vi "Build.vi"(8 "error in (no error)":errorcluster, 11 "Build in":refnum<class "AB_RESTfulWebService.lvclass">) -> (0 "error out":errorcluster, 1 "GeneratedFiles":path[](array[path]), 2 "GeneratedDirectories":path[](array[path]), 3 "Build out":refnum<class "AB_RESTfulWebService.lvclass">, 4 "GeneratedFileGUIDs":string[](array[string]), 5 "OutputDirectory":path, 7 "Dependencies":T1[](array[typedef]))   [LabVIEW 2020, in "AB_RESTfulWebService.lvclass"]
uses:
  <vilib>/AppBuilder/AB_Classes/RESTful/AB_RESTfulWebService.lvclass
  e:/builds/penguin/labview/branches/2020/dev/dist/vi.lib/AppBuilder/AB_Classes/Build/AB_Build.lvclass
  e:/builds/penguin/labview/branches/2020/dev/dist/vi.lib/AppBuilder/AB_Classes/TargetFile/AB_Targetfile.lvclass
  e:/builds/penguin/labview/branches/2020/dev/dist/vi.lib/AppBuilder/AB_Classes/WebService/AB_WebService.lvclass
  <vilib>/AppBuilder/AB_Dependency.ctl
  <vilib>/Utility/lvfile.llb/LVFileType.ctl
  <vilib>/AppBuilder/Engine/RESTful INI Generator/AB_RESTful_ServiceType.ctl
  <vilib>/AppBuilder/Engine/RESTful INI Generator/AB_RESTful_ServiceInfo.ctl
  <vilib>/AppBuilder/AB_Classes/RESTful/AB_RESTful_ServiceAttribute.ctl
  <vilib>/AppBuilder/AB_Classes/RESTful/AB_RESTful_ServiceAttributeType.ctl
  <vilib>/AppBuilder/AB_Classes/RESTful/AB_RESTfulWebService.lvclass/AB_RESTfulWebService.ctl
  <resource>/Framework/Providers/Common/provcom_StringGlobals.vi
  <vilib>/AppBuilder/AB_Classes/WebService/AB_WebService.lvclass
  <vilib>/AppBuilder/AB_Classes/Destination/AB_Destination.lvclass
  <vilib>/AppBuilder/AB_Classes/Build/AB_Build.lvclass
  <vilib>/AppBuilder/AB_Classes/TargetFile/AB_Targetfile.lvclass
  <vilib>/Utility/lvfile.llb/NI_FileType.lvlib
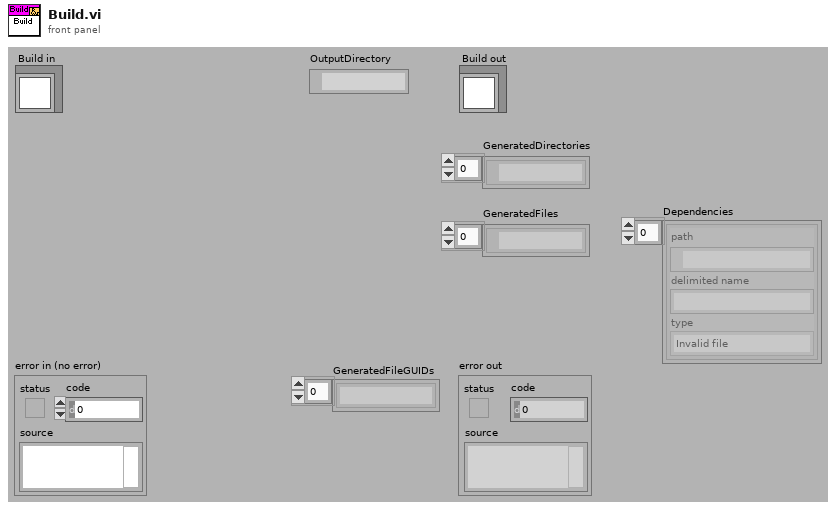
[diagram p1: front panel]
types:
  T1 = typedef "AB_Dependency.ctl" = cluster{"path":path, "delimited name":string, "type":T2}
  T2 = typedef "NI_FileType.lvlib/LVFileType.ctl" = enum32{"Invalid file", "Unknown type", "Instrument", "Control", "Polymorphic VI", "Project", "Library", "LVClass", "XControl", "XNode", "Shared library", ".NET assembly", "ActiveX interface", "CIN", "Run-time menu", "Palette menu", "Help file", "LLB", "XNode Edit Dependency", "Class Private Data Control", "Statechart", "MathScript .m file", "Ladder Diagram", "LVLibp", "XNode Build Dependency"}
  T3 = typedef "AB_RESTful_ServiceInfo.ctl" = cluster{"Service Name":string, "Web Service Library Path":path, "Server List":string[], "Debug":bool, "Service aliases":string[], "defaultStaticDoc":string, "defaultWebMethod":string, "Standalone":bool, "Service attributes":T4[], "Service Type":T6, "IniVersion":string, "MessageVersion":string, "RoutingKey":string, "Type":string, "Tags":string}
  T4 = typedef "AB_RESTful_ServiceAttribute.ctl" = cluster{"Name":string, "Service Attribute Type":T5, "Value":string}
  T5 = typedef "AB_RESTful_ServiceAttributeType.ctl" = enum32{"String", "Path"}
  T6 = typedef "AB_RESTful_ServiceType.ctl" = enum32{"RESTful", "SOAP", "AMQP"}
  T7 = typedef "AB_Build.ctl" = cluster{"buildSpecName":string, "buildSpecDescription":string, "destinations":refnum<class "AB_Destination.lvclass">[], "exclusionOption":T8, "defaultLanguage":string, "supportedLanguages":string[], "excludedDirectories":path[], "buildContext":refnum<vi>, "buildObject":T9, "preview":bool, "programatic":bool, "progressBarEvents":T10, "userLog_Path":path, "preActionID":string, "preAction_Path":path, "postActionID":string, "postAction_Path":path, "eng_checkForBrokenVIs?":bool, "eng_verboseLinkerErrors?":bool, "localDest_Path":path, "targetDest_Path":path, "removeVIObject":u16, "cache":refnum<class "PreviewCache.lvclass">, "use cache":bool, "previewCache_ID":string, "buildCache_ID":string, "eng_TempLocalDest_Path":path, "eng_collectDependencies?":bool, "versionInfo":cluster{"buildVersion":cluster{"major":u16, "minor":u16, "patch":u16, "build":u16}, "autoIncrement":bool}, "eng_enableVIChecksums":bool}
  T8 = typedef "AB_Exclusion_Option.ctl" = cluster{"typedefs":bool, "polymorphicVIs":bool, "unusedLibraryItems":bool, "modifyLibraryFile":bool, "edit-timeDependencies":bool, "inlineVIs":bool, "dependent PPLs":bool, "dependent DLLs":bool}
  T9 = typedef "ItemRef.ctl" = u64
  T10 = typedef "provcom_ProgressBar_Events.ctl" = cluster{"newJob":refnum<user-event>, "newItem":refnum<user-event>, "errorMsg":T11, "cancel":refnum<user-event>}
  T11 = typedef "mxLvBuildError.ctl" = refnum<user-event>
  T12 = typedef "AB_RESTful_RoutingTemplate.ctl" = cluster{"Template":string, "Routing Type":T13, "HTTP Method Type":T14, "VIName":string, "Default String":string, "Require API key":bool, "Auth permissions":string[], "eng_Static Alias":string, "Required Privilege":string}
  T13 = typedef "AB_RESTful_RoutingType.ctl" = enum32{"Method", "Static"}
  T14 = typedef "AB_RESTful_HTTPMethodType.ctl" = enum32{"GET", "POST", "PUT", "DELETE"}
  T15 = cluster{"Privilege":string, "Description":string, "Role":string}[]
  T16 = typedef "AB_Targetfile.ctl" = cluster{"targetfileName":string, "targetfileGUID":string, "enableDebugging":bool, "versionInfo":cluster{"productName":string, "legalCopyright":string, "companyName":string, "internalName":string, "fileDescription":string}, "eng_consolidatedTypeInfo":string, "fastFileFormat":bool, "eng_LEIFBuildData":u32, "versionIndependent":bool}
  T17 = typedef "AB_WebService.ctl" = cluster{"service aliases":string[], "standalone":bool}
  T18 = typedef "AB_Destination.ctl" = cluster{"destName":string, "path":path, "libraryName":string, "preserveHierarchy":bool, "eng_inBuild":bool, "eng_libraryReference":refnum<vi>, "eng_restictAddToNewLibrary":bool}
  T19 = typedef "AB_RESTful_Configuration.ctl" = cluster{"Service VI Type":T20, "Load VI at statup":bool, "Keep VI in memory":bool, "Output type":T21, "Output format":T22, "Use headers":bool, "Buffered":bool, "eng_Load VI by name":bool}
  T20 = typedef "AB_RESTful_VIType.ctl" = enum32{"Web Method", "Auxiliary", "eng_Internal", "eng_Content"}
  T21 = typedef "AB_RESTful_OutputType.ctl" = enum32{"Terminal", "Stream"}
  T22 = typedef "AB_RESTful_OutputFormat.ctl" = enum32{"XML", "Text", "HTML", "JSON"}
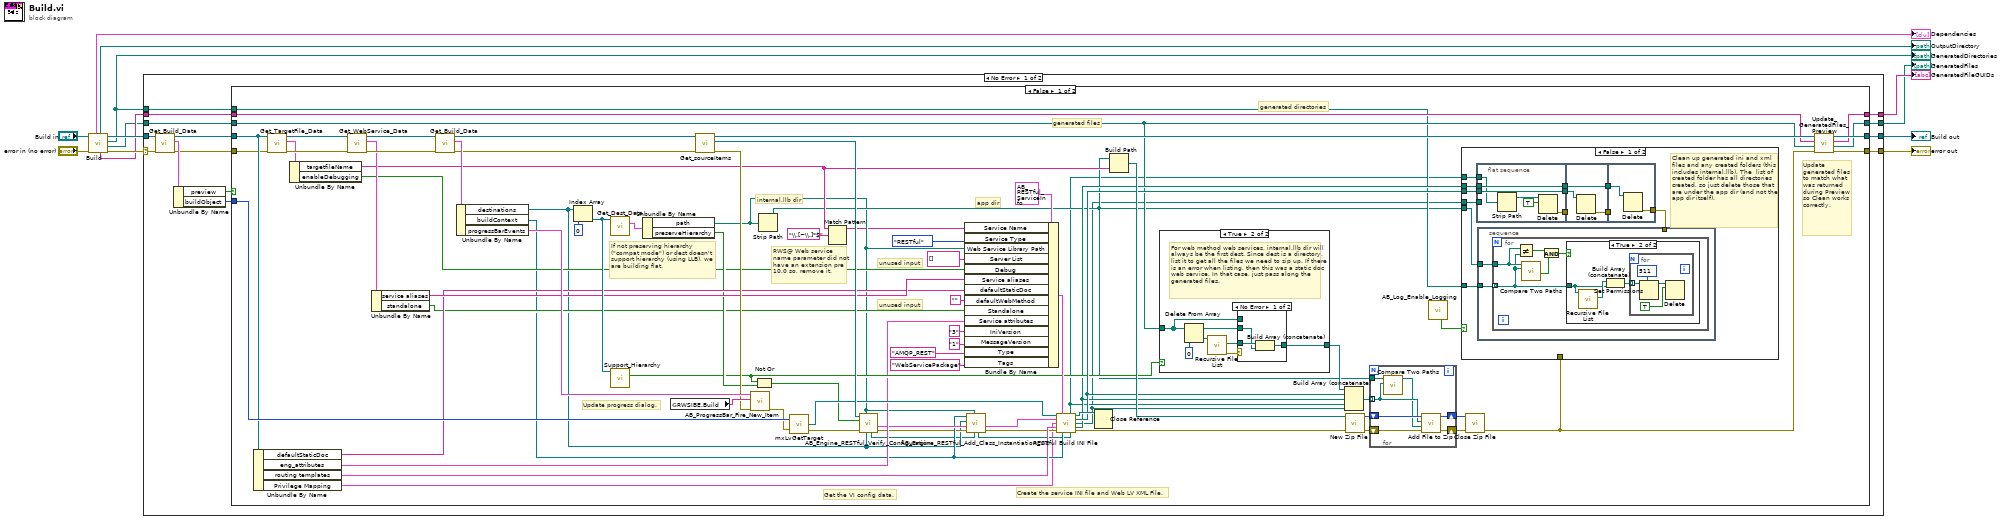
[diagram p0: block diagram]
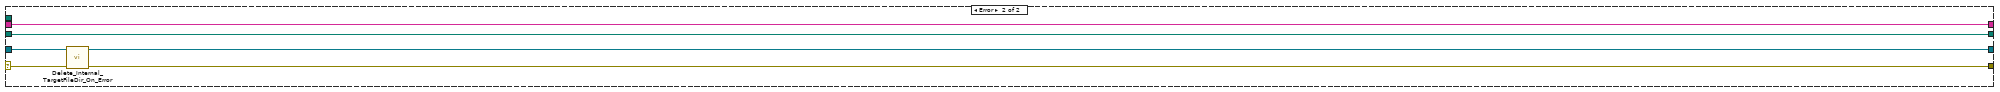
[diagram p7: hidden frame]
diagram:
  n1 = call-parent "Build.vi"("error in (no error)"="error in (no error)", "Build in"="Build in") -> ("error out"=w10:errorcluster, "GeneratedFiles"=w4:path[], "GeneratedDirectories"=w2:path[], "Build out"=w9:refnum<class "AB_RESTfulWebService.lvclass">, "GeneratedFileGUIDs"=w6:string[], "OutputDirectory"=→"OutputDirectory":path, "Dependencies"=→"Dependencies":T1[])  [unwired: 3 out]
  "GeneratedDirectories" <- w2
  n2 = case shown="No Error" w10 {
    selector: w10 -> [w25 w169]
    tunnel: w9 -> [w26 w170]
    tunnel: [w21 w167] -> w8
    tunnel: [w20 w168] -> w7
    tunnel: w4 -> [w18 w166]
    tunnel: w6 -> [w17 w165]
    tunnel: [w16 w165] -> w5
    tunnel: [w15 w166] -> w3
    tunnel: w2 -> [w14 _]
    frame No Error {
      n3 = call <vilib>:"Get_Build_Data.vi"("error in (no error)"=w25, "Class in"=w26) -> ("error out"=w23:errorcluster, "data"=w27:T7, "Class out"=w22:refnum<class "AB_RESTfulWebService.lvclass">)  [unwired: 7 out]
      n4 = Unbundle By Name(w27) -> ("preview"=w24:bool, "buildObject"=w19:T9)
      n5 = case shown="False" w24 {
        tunnel: w23 -> [w64 w163]
        tunnel: w22 -> [w66 w164]
        tunnel: [w53 w164] -> w21
        tunnel: [w55 w163] -> w20
        tunnel: w19 -> [w92 _]
        tunnel: w18 -> [w52 w162]
        tunnel: w17 -> [w51 w161]
        tunnel: [w50 w161] -> w16
        tunnel: [w49 w162] -> w15
        tunnel: w14 -> [w48 _]
        frame False {
          # "generated directories"
          # "Update generated files to match what was returned during Preview so Clean works correctly."
          # "unused input"
          # "RWS@ Web service name parameter did not have an extension pre 10.0 so, remove it."
          # "unused input"
          # "If not preserving hierarchy (\"compat mode\") or dest doesn't support hierarchy (using LLB), we are building flat."
          # "generated files"
          # "Update progress dialog."
          # "Create the service INI file and Web LV XML File."
          # "Get the VI config data."
          # "app dir"
          # "internal.llb dir"
          n6 = Unbundle By Name(w66) -> ("defaultStaticDoc"=w80:string, "eng_attributes"=w46:T4[], "routing templates"=w96:T12[], "Privilege Mapping"=w31:T15)
          n7 = call <vilib>:"Get_TargetFile_Data.vi"("error in (no error)"=w64, "AB_Targetfile in"=w66) -> ("error out"=w63:errorcluster, "data"=w62:T16, "AB_Targetfile out"=w65:refnum<class "AB_RESTfulWebService.lvclass">)  [unwired: 7 in]
          n8 = Unbundle By Name(w62) -> ("targetfileName"=w59:string, "enableDebugging"=w61:bool)
          n9 = call <vilib>:"Get_WebService_Data.vi"("error in (no error)"=w63, "Class in"=w65) -> ("error out"=w100:errorcluster, "data"=w99:T17, "class out"=w101:refnum<class "AB_RESTfulWebService.lvclass">)  [unwired: 7 out]
          n10 = Unbundle By Name(w99) -> ("service aliases"=w81:string[], "standalone"=w57:bool)
          n11 = call <vilib>:"Get_Build_Data.vi"("error in (no error)"=w100, "Class in"=w101) -> ("error out"=w84:errorcluster, "data"=w102:T7, "Class out"=w98:refnum<class "AB_RESTfulWebService.lvclass">)  [unwired: 7 out]
          n12 = Unbundle By Name(w102) -> ("destinations"=w41:refnum<class "AB_Destination.lvclass">[], "buildContext"=w44:refnum<vi>, "progressBarEvents"=w87:T10)
          n13 = Index Array(array=w41, index=0) -> (element=w82:refnum<class "AB_Destination.lvclass">)
          n14 = call <vilib>:"Get_Dest_Data.vi"("Class in"=w82) -> ("destName"=w103:T18)  [unwired: 1 in, 9 out]
          n15 = call-dynamic "Support_Hierarchy.vi"("AB_Destination in"=w82) -> ("support hierarchy"=w69:bool)  [unwired: 1 in, 9 out]
          n16 = Unbundle By Name(w103) -> ("path"=w37:path, "preserveHierarchy"=w70:bool)
          n17 = global read "provcom_StringGlobals.vi" "RWSIBE.Build"() -> (w88:string)
          n18 = call <vilib>:"Get_sourceItems.vi"("error in (no error)"=w84, "Class in"=w98) -> ("error out"=w83:errorcluster, "sourceItems"=w97:refnum<class "AB_Source.lvclass">[], "Class out"=w54:refnum<class "AB_RESTfulWebService.lvclass">)  [unwired: 7 out]
          n19 = call <vilib>:"AB_ProgressBar_Fire_New_Item.vi"("error in (no error)"=w83, "Label"=w88, "progressBarEvents in"=w87) -> ("error out"=w85:errorcluster)  [unwired: 8 out]
          n20 = Not Or(1:w70, 2:w69) -> (0:w71:bool)
          n21 = Strip Path(path=w37) -> (stripped path=w47:path)  [unwired: 1 out]
          n22 = call <resource>:"mxLvGetTarget.vi"("Item"=w92, "error in"=w85) -> ("Target"=w89:refnum<vi>, "error out"=w90:errorcluster)  [unwired: 1 out]
          n23 = Match Pattern(string=w59, regular expression="\\.[~\\.]*$") -> (before substring=w33:string)  [unwired: 4 out]
          n24 = call <vilib>:"AB_Engine_RESTful_Verify_Configuration.vi"("destinations"=w41, "path"=w37, "error in (no error)"=w90, "flat file layout"=w71, "sourceItems"=w97) -> ("error out"=w43:errorcluster, "viConfigs"=w45:T19[], "relative VI paths"=w40:path[])  [unwired: 1 in, 3 out]
          n25 = Bundle By Name(cluster=T3 {"Service Name"="", "Web Service Library Path"=path "", "Server List"=[], "Debug"=FALSE, "Service aliases"=[], "defaultStaticDoc"="", "defaultWebMethod"="", "Standalone"=FALSE, "Service attributes"=[], "Service Type"=enum."RESTful", "IniVersion"="", "MessageVersion"="", "RoutingKey"="", "Type"="", "Tags"=""} ("RESTful VI service information"), "Service Name"=w33, "Service Type"=AB_RESTful_ServiceType."RESTful", "Web Service Library Path"=w37, "Server List"=string[] [], "Debug"=w61, "Service aliases"=w81, "defaultStaticDoc"=w80, "defaultWebMethod"="", "Standalone"=w57, "Service attributes"=w46, "IniVersion"="3", "MessageVersion"="1", "Type"="AMQP_REST", "Tags"="WebServicePackage") -> (w95:T3)
          n26 = call <vilib>:"AB_Engine_RESTful_Add_Class_Instantiation_VIs.vi"("relative VI paths in"=w40, "path"=w37, "error in (no error)"=w43, "viConfigs in"=w45, "destinations"=w41, "buildContext"=w44) -> ("error out"=w42:errorcluster, "viConfigs out"=w38:T19[], "relative VI paths out"=w39:path[])  [unwired: 3 in]
          n27 = call <vilib>:"RESTful Build INI File.vi"("target reference"=w89, "RESTful VI service information"=w95, "VI Configurations"=w38, "data.Privilege Mapping"=w31, "Routing Templates"=w96, "error in (no error)"=w42, "buildContext"=w44, "relative VI paths"=w39) -> ("AMQP INI"=w36:path, "dup target reference"=w91:refnum<vi>, "INI filepath"=w74:path, "AMQP XML"=w30:path, "XML filepath"=w68:path, "error out"=w32:errorcluster)  [unwired: 2 in]
          n28 = Close Reference(reference=w91) -> ()  [unwired: 1 in, 1 out]
          n29 = Build Path(base path=w47, name or relative path=w59) -> (appended path=w75:path)
          n30 = case shown="True" w69 {
            tunnel: w52 -> [w105 w106]
            tunnel: [w105 w108] -> w72
            frame False {
            }
            frame True {
              # "For web method web services, internal.llb dir will always be the first dest. Since dest is a directory, list it to get all the files we need to zip up. If there is an error when listing, then this was a static doc web service. In that case, just pass along the generated files."
              n31 = Delete From Array(array=w106, index=0) -> (deleted portion=w111:path, array with subset deleted=w109:path[])  [unwired: 1 in]
              n32 = call <vilib>:"Recursive File List.vi"("Folder Path"=w111) -> ("error out"=w107:errorcluster, "All Files in Dir"=w110:path[])  [unwired: 2 in, 7 out]
              n33 = case shown="No Error" w107 {
                tunnel: w110 -> [w115 _]
                tunnel: w109 -> [w114 _]
                tunnel: [w113 w116] -> w108
                tunnel: w106 -> [_ w116]
                frame No Error {
                  n34 = Build Array (concatenate)(w115, w114) -> (w113:path[])
                }
                frame Error {
                }
              }
            }
          }
          n35 = Build Array (concatenate)(w72, w74, w68, w36, w30) -> (w73:path[])
          n36 = call <vilib>:"New Zip File.vi"("error in (no error)"=w32, "target"=w75) -> ("error out"=w79:errorcluster, "zip file out"=w76:i64)  [unwired: 1 in, 3 out]
          n37 = for {
            shift-right: [w122] -> w77
            shift-left: w76 -> [w123]
            shift-right: [w121] -> w78
            shift-left: w79 -> [w120]
            tunnel: w73 -> [w119] mode=indexing
            tunnel: w47 -> [w118]
            n38 = call <vilib>:"Compare Two Paths.vi"("Path 2"=w119, "Path 1"=w118) -> ("Relative Path from 1 to 2"=w117:path)  [unwired: 1 in, 8 out]
            n39 = call <vilib>:"Add File to Zip.vi"("error in (no error)"=w120, "destination path in zip"=w117, "source file path"=w119, "zip file in"=w123) -> ("error out"=w121:errorcluster, "zip file out"=w122:i64)  [unwired: 6 out]
          }
          n40 = call <vilib>:"AB_Log_Enable_Logging.vi"() -> ("keep internal.llb"=w86:bool)  [unwired: 2 in, 9 out]
          n41 = call <vilib>:"Close Zip File.vi"("error in (no error)"=w78, "zip file in"=w77) -> ("error out"=w56:errorcluster)  [unwired: 1 in, 4 out]
          n42 = case shown="False" w86 {
            tunnel: w74 -> [w135 _]
            tunnel: w56 -> [_ _]
            tunnel: w68 -> [w133 _]
            tunnel: w48 -> [w131 _]
            tunnel: w47 -> [w130 _]
            tunnel: w36 -> [w129 _]
            tunnel: w30 -> [w126 _]
            frame False {
              # "Clean up generated ini and xml files and any created folders (this includes internal.llb). The  list of created folder has all directories created, so just delete those that are under the app dir (and not the app dir itself)."
              n43 = flat-sequence {
                tunnel: w129 -> [w136]
                tunnel: w133 -> [w140]
                tunnel: w135 -> [w141]
                tunnel: [w141] -> w128
                tunnel: [w140] -> w127
                tunnel: w126 -> [_]
                tunnel: [w139] -> w125
                tunnel: [w144] -> w134
                tunnel: [w143] -> w132
                tunnel: w128 -> [w142]
                tunnel: w127 -> [w143]
                tunnel: w125 -> [_]
                tunnel: w134 -> [_]
                tunnel: w132 -> [w146]
                tunnel: [w145] -> w124
                frame #0 {
                  n44 = Strip Path(path=w136) -> (stripped path=w138:path)  [unwired: 1 out]
                  n45 = Delete(path (use dialog)=w138, entire hierarchy (F)=TRUE) -> (error out=w139:errorcluster)  [unwired: 1 in, 4 out]
                }
                frame #1 {
                  n46 = Delete(path (use dialog)=w142) -> (error out=w144:errorcluster)  [unwired: 2 in, 4 out]
                }
                frame #2 {
                  n47 = Delete(path (use dialog)=w146) -> (error out=w145:errorcluster)  [unwired: 2 in, 4 out]
                }
              }
              n48 = stacked-sequence {
                tunnel: w131 -> [w148]
                tunnel: w130 -> [w147]
                tunnel: w124 -> [_]
                frame #0 {
                  n49 = for {
                    tunnel: w148 -> [w152] mode=indexing
                    tunnel: w147 -> [w153]
                    n50 = Not Equal?(x=w153, y=w152) -> (x != y?=w151:bool)
                    n51 = call <vilib>:"Compare Two Paths.vi"("Path 2"=w152, "Path 1"=w153) -> ("Path 2 Relative to Path 1?"=w150:bool)  [unwired: 1 in, 8 out]
                    n52 = And(x=w151, y=w150) -> (x .and. y?=w149:bool)
                    n53 = case shown="True" w149 {
                      tunnel: w152 -> [_ w154]
                      frame False {
                      }
                      frame True {
                        n54 = call <vilib>:"Recursive File List.vi"("Folder Path"=w154) -> ("All Files in Dir"=w156:path[])  [unwired: 2 in, 8 out]
                        n55 = Build Array (concatenate)(w156, w154) -> (w155:path[])
                        n56 = for {
                          tunnel: w155 -> [w157] mode=indexing
                          n57 = Set Permissions(7:i16 511 ("permissions"), 11:w157) -> (3:w158:path)  [unwired: 1 in, 3 out]
                          n58 = Delete(path (use dialog)=w158, entire hierarchy (F)=TRUE) -> ()  [unwired: 1 in, 5 out]
                        }
                      }
                    }
                  }
                }
              }
            }
            frame True {
            }
          }
          n59 = call-dynamic "Update_GeneratedFiles_Preview.vi"("error in (no error)"=w56, "GeneratedFiles in"=w52, "GeneratedFileGUIDs in"=w51, "Build in"=w54) -> ("error out"=w55:errorcluster, "GeneratedFiles out"=w49:path[], "GeneratedFileGUIDs out"=w50:string[], "Build out"=w53:refnum<class "AB_RESTfulWebService.lvclass">)  [unwired: 4 in]
        }
        frame True {
        }
      }
    }
    frame Error {
      n60 = call-dynamic "Delete_Internal_TargetFileDir_On_Error.vi"("error in (no error)"=w169, "Build in"=w170) -> ("error out"=w168:errorcluster, "Build out"=w167:refnum<class "AB_RESTfulWebService.lvclass">)  [unwired: 8 in]
    }
  }
  "error out" <- w7
  "Build out" <- w8
  "GeneratedFiles" <- w3
  "GeneratedFileGUIDs" <- w5
